vi "Write to Data Source.vi"(8 "error in (no error)":errorcluster, 11 "INI in":refnum<class "Projects-INI.lvclass">) -> (0 "error out":errorcluster, 3 "INI out":refnum<class "Projects-INI.lvclass">)   [LabVIEW 2020, in "Projects-INI.lvclass"]
doc: "Write the data currently in the Project class data to the data source.\n\n03/2025 Erich Schlieper"
uses:
  Projects-INI.lvclass
  C:/Apps/LVTimeTracker/LVTimeTracker/Projects/Parent/Projects.lvclass
  Projects-INI.lvclass/Projects-INI.ctl
  <vilib>/Utility/config.llb/Write Key (String).vi
  <vilib>/Utility/config.llb/NI_LVConfig.lvlib
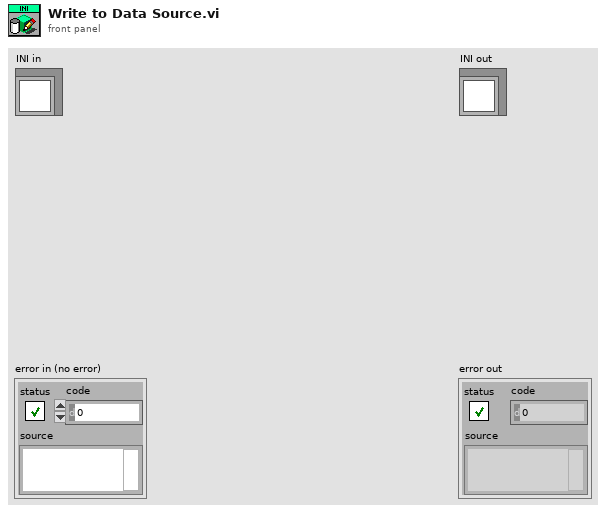
[diagram p1: front panel]
types:
  T1 = typedef "Project Info.ctl" = cluster{"Project Active?":bool, "Tasks":set{string}, "Task Active":map{string, bool}}
  T2 = typedef "NI_LVConfig.lvlib/Config Data RefNum.ctl" = refnum<k1>
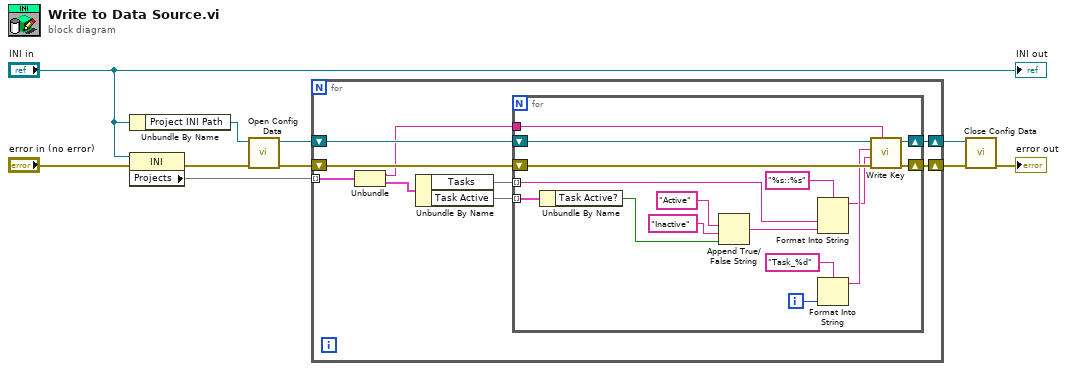
[diagram p0: block diagram]
diagram:
  n1 = Unbundle By Name("INI in") -> ("Project INI Path"=w8:path)
  n2 = property class="INI"(reference="INI in", error in="error in (no error)") -> (error out=w9:errorcluster, "Projects"=w5:map{string, T1})  [unwired: 1 out]
  n3 = call <vilib>:"Open Config Data.vi"("error in (no error)"=w9, "configuration file path"=w8) -> ("error out"=w6:errorcluster, "refnum"=w7:T2)  [unwired: 7 in, 1 out]
  n4 = for {
    tunnel: w5 -> [w17] mode=indexing
    shift-right: [w14] -> w1
    shift-left: w7 -> [w19]
    shift-right: [w13] -> w3
    shift-left: w6 -> [w18]
    n5 = Unbundle(w17) -> (w15:string, "Project Info"=w16:T1)
    n6 = Unbundle By Name(w16) -> ("Tasks"=w12:set{string}, "Task Active"=w11:map{string, bool})
    n7 = for {
      tunnel: w12 -> [w26] mode=indexing
      tunnel: w15 -> [w33]
      shift-right: [w29] -> w14
      shift-left: w19 -> [w35]
      shift-right: [w28] -> w13
      shift-left: w18 -> [w34]
      tunnel: w11 -> [w25] mode=indexing
      i -> [w32]
      n8 = Unbundle By Name(w25) -> ("Task Active?"=w24:bool)
      n9 = Append True/False String(1:w24, 2:"Inactive" ("true string"), 3:"Active" ("true string")) -> (0:w23:string)  [unwired: 1 in]
      n10 = Format Into String(format string="%s::%s", w26, w23) -> (resulting string=w20:string)  [unwired: 2 in, 1 out]
      n11 = Format Into String(format string="Task_%d", w32) -> (resulting string=w30:string)  [unwired: 2 in, 1 out]
      n12 = call-poly <vilib>:"Write Key.vi"("section"=w33, "error in (no error)"=w34, "value"=w20, "key"=w30, "refnum"=w35) -> ("error out"=w28:errorcluster, "refnum out"=w29:T2)  [unwired: 4 in, 1 out]
    }
  }
  n13 = call <vilib>:"Close Config Data.vi"("error in (no error)"=w3, "refnum"=w1) -> ("error out"=→"error out":errorcluster)  [unwired: 8 in, 1 out]
  "INI out" <- "INI in"
